vi "Agilent 532XX Series Acquire Frequency.vi"() -> ()   [LabVIEW 2024]
doc: "This example shows how to acquire frequency using the VIs of the driver.\n\n<B>Note:</B> This example is available only on the Agilent 53220A/53230A."
uses:
  Public/Configure/Measurement/Configure Measurement (Frequency).vi
  Public/Data/Read Measurement (Single).vi
  Agilent 532XX Series.lvlib
panel:
  in  "Gate Stop Slop (1: Negative)":i32(ring)=1 items=["Positive", "Negative"]
  in  "Gate Stop Source (0:  Immediate)":i32(ring) items=[" Immediate", " External"]
  in  "Gate Stop Holdoff Event (1)":dbl=1.0
  in  "Gate Stop Holdoff Source (1: Time)":i32(ring)=1 items=[" Immediate", "Time", "Events"]
  in  "Gate Start Delay Time (0 s)":dbl
  in  "Gate Start Delay Source (1: Time)":i32(ring)=1 items=["Immediate", "Time", " Events "]
  in  "Gate Start Slop (1: Negative)":i32(ring)=1 items=["Positive", "Negative"]
  in  "Gate Start Source (0: Immediate)":i32(ring) items=["Immediate", "External"]
  in  "Gate Source (0: Time)":i32(ring) items=["Time", "External", "Input1", "Input2", "Advanced"]
  in  "Gate External Source (0: BNC)":i32(ring) items=["BNC", "Input 1", "Input 2"]
  in  "Timeout (10000 ms)":u32=10000
  out "Frequency":dbl format="%#_12g"
  in  "VISA resource name":refnum<visa-resource-name>
  # "(c) 2010-2015 National Instruments.  ALL RIGHTS RESERVED."
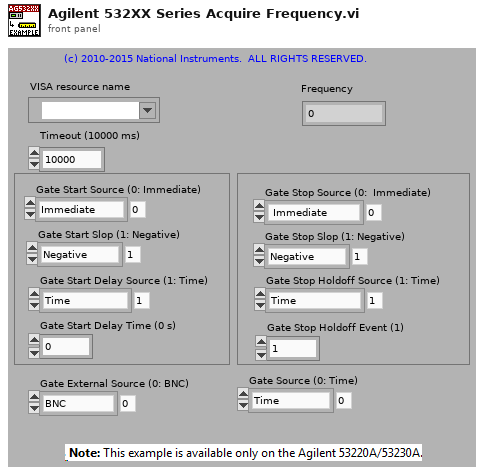
[diagram p1: front panel]
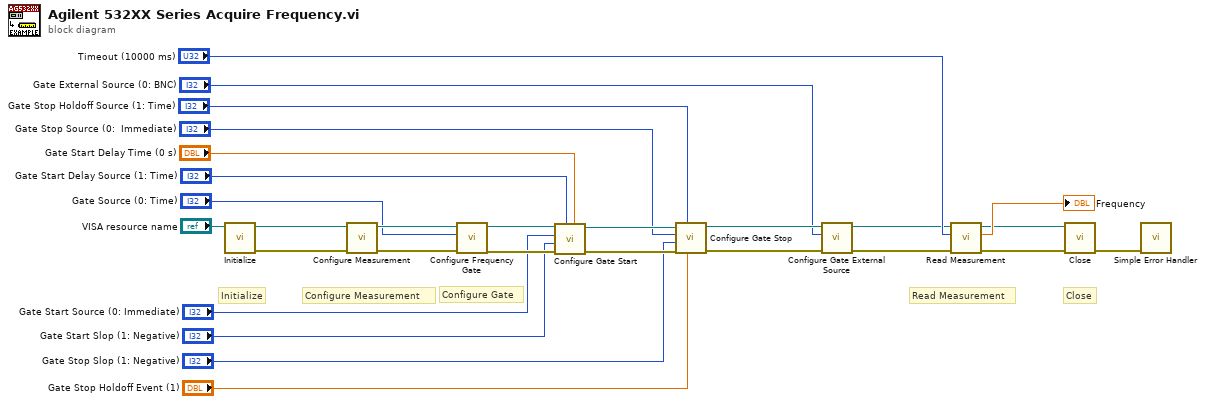
[diagram p0: block diagram]
diagram:
  # "Configure Gate"
  # "Close"
  # "Read Measurement"
  # "Initialize"
  # "Configure Measurement"
  n1 = call "Initialize.vi"("VISA resource name"="VISA resource name") -> ("error out"=w25:errorcluster, "VISA resource name out"=w26:refnum<visa-resource-name>)  [unwired: 3 in, 6 out]
  n2 = call-poly "Configure Measurement.vi"("error in (no error)"=w25, "VISA resource name"=w26) -> ("error out"=w13:errorcluster, "VISA resource name out"=w12:refnum<visa-resource-name>)  [unwired: 3 in, 5 out]
  n3 = call "Configure Frequency Gate.vi"("error in (no error)"=w13, "Gate Source (0: Time)"="Gate Source (0: Time)", "VISA resource name"=w12) -> ("error out"=w14:errorcluster, "VISA resource name out"=w11:refnum<visa-resource-name>)  [unwired: 3 in, 4 out]
  n4 = call "Configure Gate Start.vi"("Gate Start Delay Time (0 s)"="Gate Start Delay Time (0 s)", "Gate Start Delay Source (1: Time)"="Gate Start Delay Source (1: Time)", "error in (no error)"=w14, "Gate Start Slop (1: Negative)"="Gate Start Slop (1: Negative)", "Gate Start Source (0: Immediate)"="Gate Start Source (0: Immediate)", "VISA resource name"=w11) -> ("error out"=w15:errorcluster, "VISA resource name out"=w16:refnum<visa-resource-name>)  [unwired: 1 in, 3 out]
  n5 = call "Configure Gate Stop.vi"("Gate Stop Holdoff Event (1)"="Gate Stop Holdoff Event (1)", "Gate Stop Holdoff Source (1: Time)"="Gate Stop Holdoff Source (1: Time)", "error in (no error)"=w15, "Gate Stop Slop (1: Negative)"="Gate Stop Slop (1: Negative)", "Gate Stop Source (0:  Immediate)"="Gate Stop Source (0:  Immediate)", "VISA resource name"=w16) -> ("error out"=w17:errorcluster, "VISA resource name out"=w18:refnum<visa-resource-name>)  [unwired: 1 in, 3 out]
  n6 = call "Configure Gate External Source.vi"("error in (no error)"=w17, "Gate External Source (0: BNC)"="Gate External Source (0: BNC)", "VISA resource name"=w18) -> ("error out"=w19:errorcluster, "VISA resource name out"=w20:refnum<visa-resource-name>)  [unwired: 7 out]
  n7 = call-poly "Read Measurement.vi"("error in (no error)"=w19, "Timeout (10000 ms)"="Timeout (10000 ms)", "VISA resource name"=w20) -> ("error out"=w23:errorcluster, "Measurement"=→"Frequency":dbl, "VISA resource name out"=w21:refnum<visa-resource-name>)  [unwired: 6 out]
  n8 = call "Close.vi"("error in (no error)"=w23, "VISA resource name"=w21) -> ("error out"=w27:errorcluster)  [unwired: 9 out]
  n9 = call <vilib>:"Simple Error Handler.vi"("error in (no error)"=w27) -> ()  [unwired: 1 in, 8 out]
